vi "Multiple Roots Visualization.vi"() -> ()   [LabVIEW 2016, in "Tree Manager.lvclass"]
uses:
  Tree Manager.lvclass
panel:
  out "All Names":string[](array[string])
  out "All IDs":string[](array[string])
  out "Roots Names":string[](array[string])
  out "Roots IDs":string[](array[string])
  in  "Tree 2":string(tree)
  in  "Tree":string(tree)
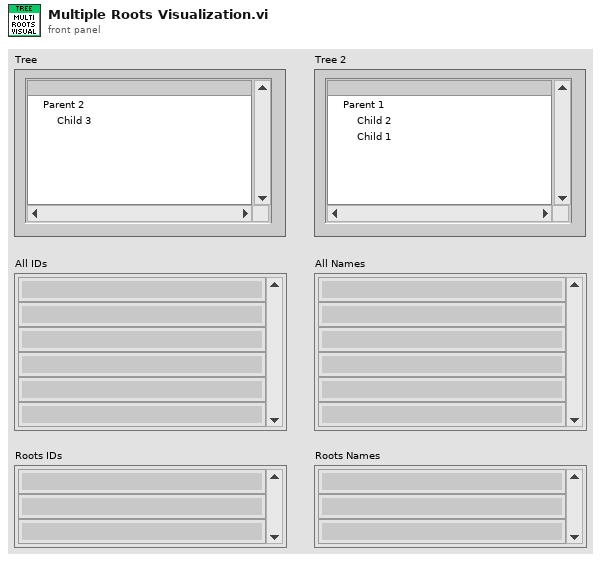
[diagram p1: front panel]
types:
  T1 = typedef "Tree Manager.lvclass/Session Handle.ctl" = refnum<data-value>
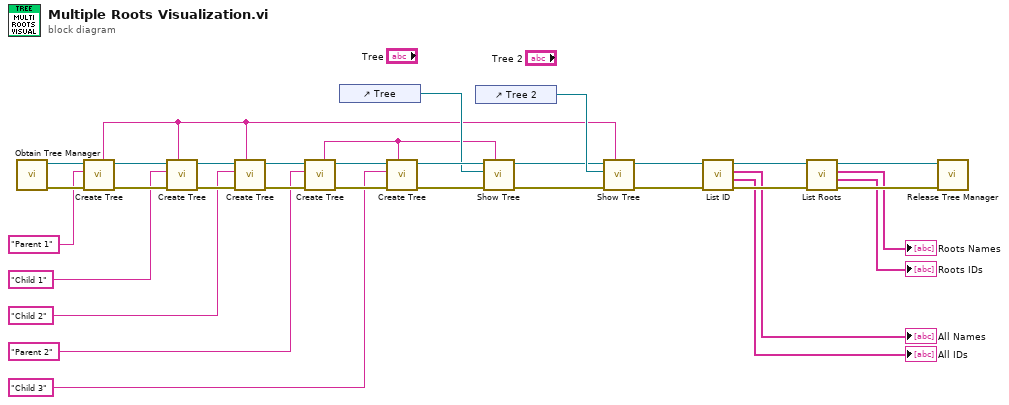
[diagram p0: block diagram]
diagram:
  n1 = call "Obtain Tree Manager.vi"() -> ("Error Out"=w32:errorcluster, "Tree Manager"=w33:T1)  [unwired: 10 in]
  n2 = call "Create Tree.vi"("Error In"=w32, "Name"="Parent 1", "Tree Manager"=w33) -> ("Error Out"=w30:errorcluster, "Tree Manager"=w31:T1, "Unique ID"=w2:string)  [unwired: 6 in]
  n3 = call "Create Tree.vi"("Parent ID (empty)"=w2, "Error In"=w30, "Name"="Child 1", "Tree Manager"=w31) -> ("Error Out"=w28:errorcluster, "Tree Manager"=w29:T1)  [unwired: 5 in, 1 out]
  n4 = call "Create Tree.vi"("Parent ID (empty)"=w2, "Error In"=w28, "Name"="Child 2", "Tree Manager"=w29) -> ("Error Out"=w26:errorcluster, "Tree Manager"=w27:T1)  [unwired: 5 in, 1 out]
  n5 = call "Create Tree.vi"("Error In"=w26, "Name"="Parent 2", "Tree Manager"=w27) -> ("Error Out"=w24:errorcluster, "Tree Manager"=w25:T1, "Unique ID"=w1:string)  [unwired: 6 in]
  n6 = control-ref of="Tree"() -> (w16:refnum<vi>)
  n7 = call "Create Tree.vi"("Parent ID (empty)"=w1, "Error In"=w24, "Name"="Child 3", "Tree Manager"=w25) -> ("Error Out"=w22:errorcluster, "Tree Manager"=w23:T1)  [unwired: 5 in, 1 out]
  n8 = control-ref of="Tree 2"() -> (w17:refnum<vi>)
  n9 = call "Show Tree.vi"("Root ID"=w1, "Error In"=w22, "Tree Ref"=w16, "Tree Manager"=w23) -> ("Error Out"=w10:errorcluster, "Tree Manager"=w11:T1)  [unwired: 6 in]
  n10 = call "Show Tree.vi"("Root ID"=w2, "Error In"=w10, "Tree Ref"=w17, "Tree Manager"=w11) -> ("Error Out"=w6:errorcluster, "Tree Manager"=w9:T1)  [unwired: 6 in]
  n11 = call "List ID.vi"("Error In"=w6, "Tree Manager"=w9) -> ("Error Out"=w7:errorcluster, "Child IDs"=→"All IDs":string[], "Child Names"=→"All Names":string[], "Tree Manager"=w8:T1)  [unwired: 6 in]
  n12 = call "List Roots.vi"("Error In"=w7, "Tree Manager"=w8) -> ("Error Out"=w15:errorcluster, "Roots IDs"=→"Roots IDs":string[], "Roots Names"=→"Roots Names":string[], "Tree Manager"=w14:T1)  [unwired: 6 in]
  n13 = call "Release Tree Manager.vi"("Error In"=w15, "Tree Manager"=w14) -> ()  [unwired: 9 in, 1 out]
